vi "6 (SubVI).vi"(10 "Scalar":dbl, 11 "Digital in":refnum<vi>) -> (3 "Cluster":cluster{dbl[], dbl[]})   [LabVIEW 2020]
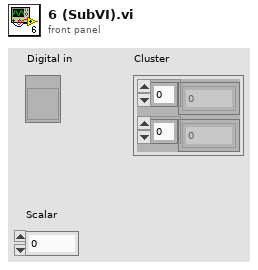
[diagram p1: front panel]
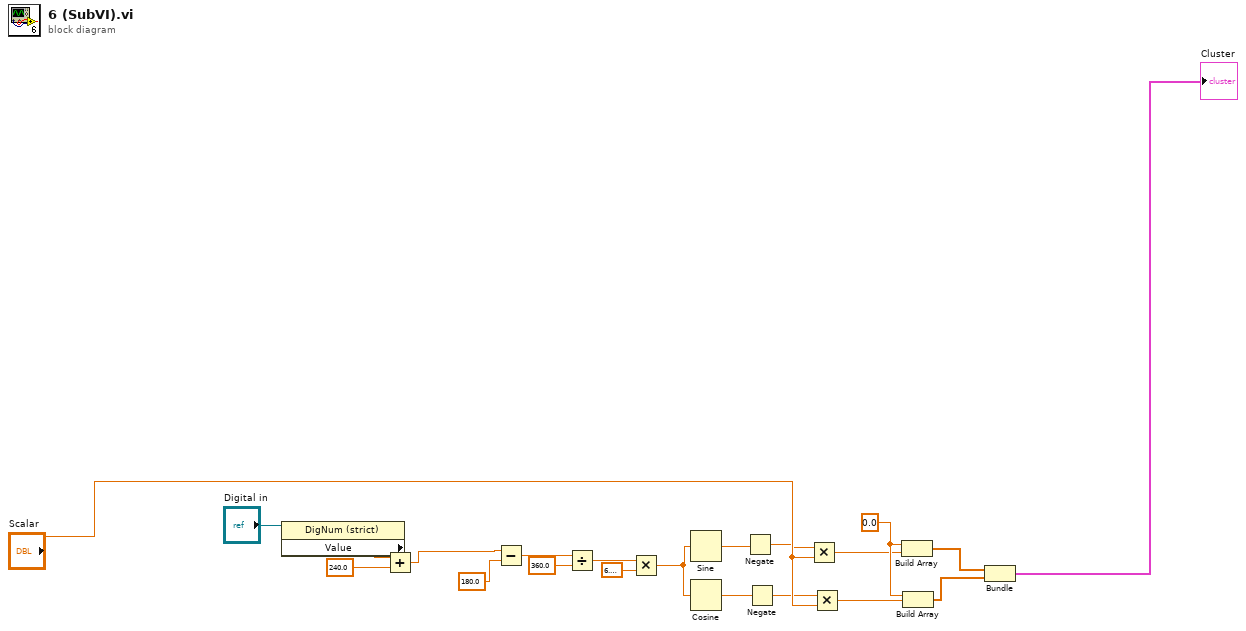
[diagram p0: block diagram]
diagram:
  w14 = 0.0 ("element")
  n1 = property class="DigNum (strict)"(reference="Digital in") -> ("Value"=w19:dbl)  [unwired: 1 in, 2 out]
  n2 = Add(x=w19, y=240.0) -> (x+y=w21:dbl)
  n3 = Subtract(x=w21, y=180.0) -> (x-y=w3:dbl)
  n4 = Divide(x=w3, y=360.0) -> (x/y=w5:dbl)
  n5 = Multiply(x=w5, y=6.283185307179586) -> (x*y=w7:dbl)
  n6 = Sine(x=w7) -> (sin(x)=w8:dbl)
  n7 = Cosine(x=w7) -> (cos(x)=w9:dbl)
  n8 = Negate(x=w8) -> (-x=w11:dbl)
  n9 = Negate(x=w9) -> (-x=w10:dbl)
  n10 = Multiply(x=w11, y="Scalar") -> (x*y=w13:dbl)
  n11 = Multiply(x=w10, y="Scalar") -> (x*y=w12:dbl)
  n12 = Build Array(w14, w13) -> (w15:dbl[])
  n13 = Build Array(w14, w12) -> (w16:dbl[])
  n14 = Bundle(w15, w16) -> (→"Cluster":cluster{dbl[], dbl[]})  [unwired: 1 in]
